vi "Check and Remove Current Row Status.vi"(1 "Row":i32, 2 "Active Positions":bool[](array[boolean]), 3 "Rack Status In":bool[](array[boolean])) -> (0 "Rack Status Out":bool[](array[boolean]))   [LabVIEW 2021]
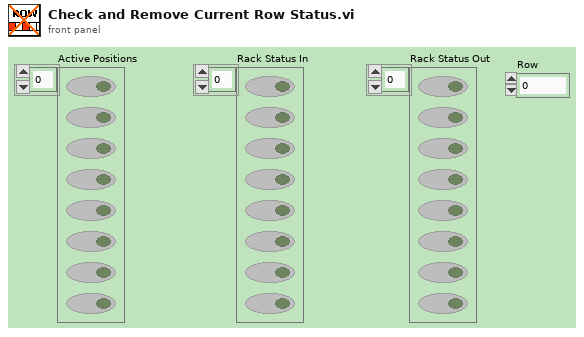
[diagram p1: front panel]
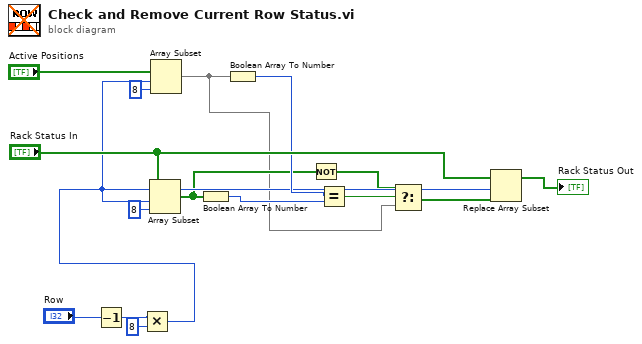
[diagram p0: block diagram]
diagram:
  n1 = Decrement(x="Row") -> (x-1=w11:i32)
  n2 = Multiply(x=w11, y=8) -> (x*y=w4:i32)
  n3 = Array Subset(array="Rack Status In", index=w4, length=8) -> (w3:bool[])
  n4 = Array Subset(array="Active Positions", index=w4, length=8) -> (w1:bool[])
  n5 = Boolean Array To Number(Boolean array=w3) -> (number=w8:u32)
  n6 = Boolean Array To Number(Boolean array=w1) -> (number=w7:u32)
  n7 = Not(x=w3) -> (.not. x?=w2:bool[])
  n8 = Equal?(x=w7, y=w8) -> (x = y?=w9:bool)
  n9 = Select(t=w2, s=w9, f=w1) -> (s? t:f=w14:bool[])
  n10 = Replace Array Subset(array="Rack Status In", new element=w14, index=w4) -> (→"Rack Status Out":bool[])
